vi "Check For Updates.vi"(0 "GUI search key":string="###GUI_HARP_CAMERA_CONTROLLER###", 2 "shortcut key":string, 13 "timeout (days)":dbl=1.0) -> (8 "check for updates":bool)   [LabVIEW 2010]
uses:
  <vilib>/Utility/sysdir.llb/System Directory Type.ctl
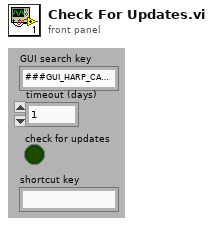
[diagram p1: front panel]
types:
  T1 = typedef "System Directory Type.ctl" = i32
  T2 = enum16{"open", "replace", "create", "open or create", "replace or create", "replace or create with confirmation"}
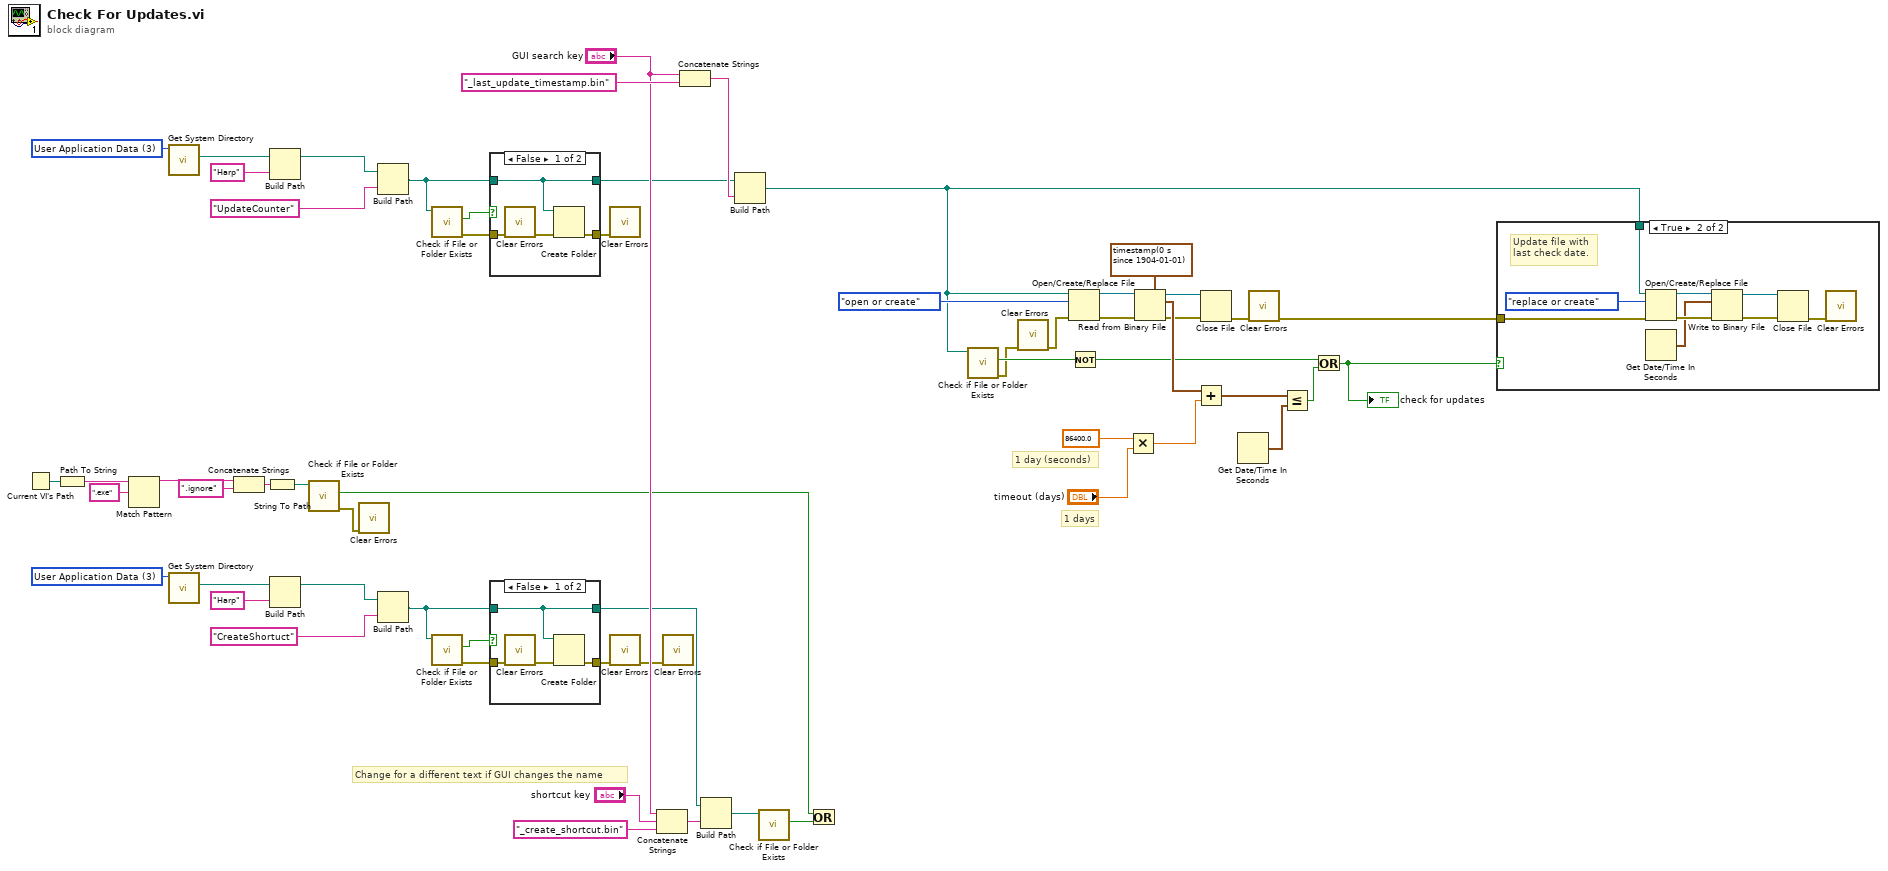
[diagram p0: block diagram]
diagram:
  w18 = T1 3 items=["User Home"=0, "User Desktop"=1, "User Documents"=2, "User Application Data"=3, "User Preferences"=4, "User Temporary"=5, "Public Documents"=6, "Public Application Data"=7, "Public Preferences"=8, "Public Cache"=13, "System Core Libraries"=9, "System Installed Libraries"=10, "Application Files"=11, "Boot Volume Root"=12] ("system directory type")
  w31 = T1 3 items=["User Home"=0, "User Desktop"=1, "User Documents"=2, "User Application Data"=3, "User Preferences"=4, "User Temporary"=5, "Public Documents"=6, "Public Application Data"=7, "Public Preferences"=8, "Public Cache"=13, "System Core Libraries"=9, "System Installed Libraries"=10, "Application Files"=11, "Boot Volume Root"=12] ("system directory type")
  # "Change for a different text if GUI changes the name"
  # "1 days"
  # "1 day (seconds)"
  n1 = Current VI's Path() -> (path=w8:path)
  n2 = Path To String(path=w8) -> (string=w9:string)
  n3 = Match Pattern(string=w9, regular expression=".exe") -> (before substring=w10:string)  [unwired: 1 in, 3 out]
  n4 = call <vilib>:"Get System Directory.vi"("system directory type"=w31) -> ("system directory"=w30:path)  [unwired: 10 in]
  n5 = call <vilib>:"Get System Directory.vi"("system directory type"=w18) -> ("system directory"=w19:path)  [unwired: 10 in]
  n6 = Concatenate Strings(w10, ".ignore" ("name or relative path")) -> (w6:string)
  n7 = String To Path(string=w6) -> (path=w4:path)
  n8 = Build Path(base path=w30, name or relative path="Harp") -> (appended path=w29:path)
  n9 = Build Path(base path=w19, name or relative path="Harp") -> (appended path=w20:path)
  n10 = call <vilib>:"Check if File or Folder Exists.vi"("path"=w4) -> ("error out"=w2:errorcluster, "file or folder exists?"=w3:bool)  [unwired: 8 in, 1 out]
  n11 = call <vilib>:"Clear Errors.vi"("error in (no error)"=w2) -> ()  [unwired: 6 in, 1 out]
  n12 = Build Path(base path=w29, name or relative path="UpdateCounter") -> (appended path=w32:path)
  n13 = Build Path(base path=w20, name or relative path="CreateShortuct") -> (appended path=w17:path)
  n14 = call <vilib>:"Check if File or Folder Exists.vi"("path"=w32) -> ("error out"=w35:errorcluster, "file or folder exists?"=w33:bool)  [unwired: 8 in, 1 out]
  n15 = call <vilib>:"Check if File or Folder Exists.vi"("path"=w17) -> ("error out"=w14:errorcluster, "file or folder exists?"=w16:bool)  [unwired: 8 in, 1 out]
  n16 = case shown="False" w33 {
    tunnel: w32 -> [w60 w64]
    tunnel: w35 -> [w63 w65]
    tunnel: [w61 w65] -> w34
    tunnel: [w60 w64] -> w11
    frame False {
      n17 = call <vilib>:"Clear Errors.vi"("error in (no error)"=w63) -> ("error out"=w62:errorcluster)  [unwired: 6 in]
      n18 = Create Folder(path (use dialog)=w60, error in=w62) -> (error out=w61:errorcluster)  [unwired: 1 in, 2 out]
    }
    frame True {
    }
  }
  n19 = case shown="False" w16 {
    tunnel: w17 -> [w66 w70]
    tunnel: w14 -> [w69 w71]
    tunnel: [w67 w71] -> w15
    tunnel: [w66 w70] -> w12
    frame False {
      n20 = call <vilib>:"Clear Errors.vi"("error in (no error)"=w69) -> ("error out"=w68:errorcluster)  [unwired: 6 in]
      n21 = Create Folder(path (use dialog)=w66, error in=w68) -> (error out=w67:errorcluster)  [unwired: 1 in, 2 out]
    }
    frame True {
    }
  }
  n22 = call <vilib>:"Clear Errors.vi"("error in (no error)"=w34) -> ()  [unwired: 6 in, 1 out]
  n23 = call <vilib>:"Clear Errors.vi"("error in (no error)"=w15) -> ("error out"=w1:errorcluster)  [unwired: 6 in]
  n24 = Concatenate Strings("GUI search key", "shortcut key", "_create_shortcut.bin" ("name or relative path")) -> (w27:string)
  n25 = call <vilib>:"Clear Errors.vi"("error in (no error)"=w1) -> ()  [unwired: 6 in, 1 out]
  n26 = Concatenate Strings("GUI search key", "_last_update_timestamp.bin" ("name or relative path")) -> (w37:string)
  n27 = Build Path(base path=w12, name or relative path=w27) -> (appended path=w22:path)
  n28 = Build Path(base path=w11, name or relative path=w37) -> (appended path=w45:path)
  n29 = call <vilib>:"Check if File or Folder Exists.vi"("path"=w22) -> ("file or folder exists?"=w23:bool)  [unwired: 8 in, 2 out]
  n30 = Or(x=w3, y=w23) -> ()  [unwired: 1 out]
  n31 = call <vilib>:"Check if File or Folder Exists.vi"("path"=w45) -> ("error out"=w41:errorcluster, "file or folder exists?"=w44:bool)  [unwired: 8 in, 1 out]
  n32 = call <vilib>:"Clear Errors.vi"("error in (no error)"=w41) -> ("error out"=w40:errorcluster)  [unwired: 6 in]
  n33 = Open/Create/Replace File(file path (use dialog)=w45, error in=w40, operation (0:open)=T2."open or create") -> (refnum out=w56:refnum<file>, error out=w57:errorcluster)  [unwired: 3 in, 1 out]
  n34 = Not(x=w44) -> (.not. x?=w42:bool)
  n35 = Multiply(x=86400.0 ("y"), y="timeout (days)") -> (x*y=w39:dbl)
  n36 = Read from Binary File(5:timestamp(0 s since 1904-01-01) ("current time"), 8:w57, 11:w56) -> (0:w50:errorcluster, 2:w53:timestamp, 3:w49:refnum<file>)  [unwired: 3 in, 1 out]
  n37 = Add(x=w53, y=w39) -> (x+y=w52:timestamp)
  n38 = Close File(refnum=w49, error in=w50) -> (error out=w48:errorcluster)  [unwired: 1 out]
  n39 = Get Date/Time In Seconds() -> (seconds since 1Jan1904=w51:timestamp)
  n40 = call <vilib>:"Clear Errors.vi"("error in (no error)"=w48) -> ("error out"=w47:errorcluster)  [unwired: 6 in]
  n41 = Less Or Equal?(x=w52, y=w51) -> (x <= y?=w46:bool)
  n42 = Or(x=w42, y=w46) -> (x .or. y?=w43:bool)
  "check for updates" <- w43
  n43 = case shown="True" w43 {
    tunnel: w45 -> [_ w75]
    tunnel: w47 -> [_ w74]
    frame False {
    }
    frame True {
      # "Update file with\nlast check date."
      n44 = Open/Create/Replace File(file path (use dialog)=w75, error in=w74, operation (0:open)=T2."replace or create") -> (refnum out=w78:refnum<file>, error out=w77:errorcluster)  [unwired: 3 in, 1 out]
      n45 = Get Date/Time In Seconds() -> (seconds since 1Jan1904=w73:timestamp)
      n46 = Write to Binary File(file (use dialog)=w78, data=w73, error in=w77) -> (refnum out=w80:refnum<file>, error out=w79:errorcluster)  [unwired: 3 in, 1 out]
      n47 = Close File(refnum=w80, error in=w79) -> (error out=w72:errorcluster)  [unwired: 1 out]
      n48 = call <vilib>:"Clear Errors.vi"("error in (no error)"=w72) -> ()  [unwired: 6 in, 1 out]
    }
  }
